vi "Fault_Abnormal_state.vi"() -> ()   [LabVIEW 2016]
panel:
  in  "e_MGCC_UnPlanISD_error":errorcluster
  in  "e_MGCC_PlanISD_error":errorcluster
  in  "Abnormal state flag":bool[](array[boolean])
  in  "Fault state flag":bool[](array[boolean])
  out "e_MGCC_StaEst_error":errorcluster[](array[cluster])
  out "e_MGCC_Resync_error":errorcluster[](array[cluster])
  out "e_MGCC_PQBal_error":errorcluster[](array[cluster])
  out "e_MGCC_PVFcst_error":errorcluster[](array[cluster])
  out "e_MGCC_ProtCoord_error":errorcluster[](array[cluster])
  out "e_MGCC_MdlMgmt_error":errorcluster
  out "e_MGCC_LoadFcst_error":errorcluster[](array[cluster])
  out "e_MGCC_Datalog_error":errorcluster[](array[cluster])
  out "e_MGCC_FntStaMach_error":errorcluster
  out "e_MGCC_EnergyMgmt_error":errorcluster[](array[cluster])
  out "e_MGCC_Commun_error":errorcluster[](array[cluster])
  out "e_MGCC_BlkStart_error":errorcluster[](array[cluster])
  out "Function enable by fault/abnormal":bool[][](array[boolean])
  out "Error State":errorcluster[](array[cluster])
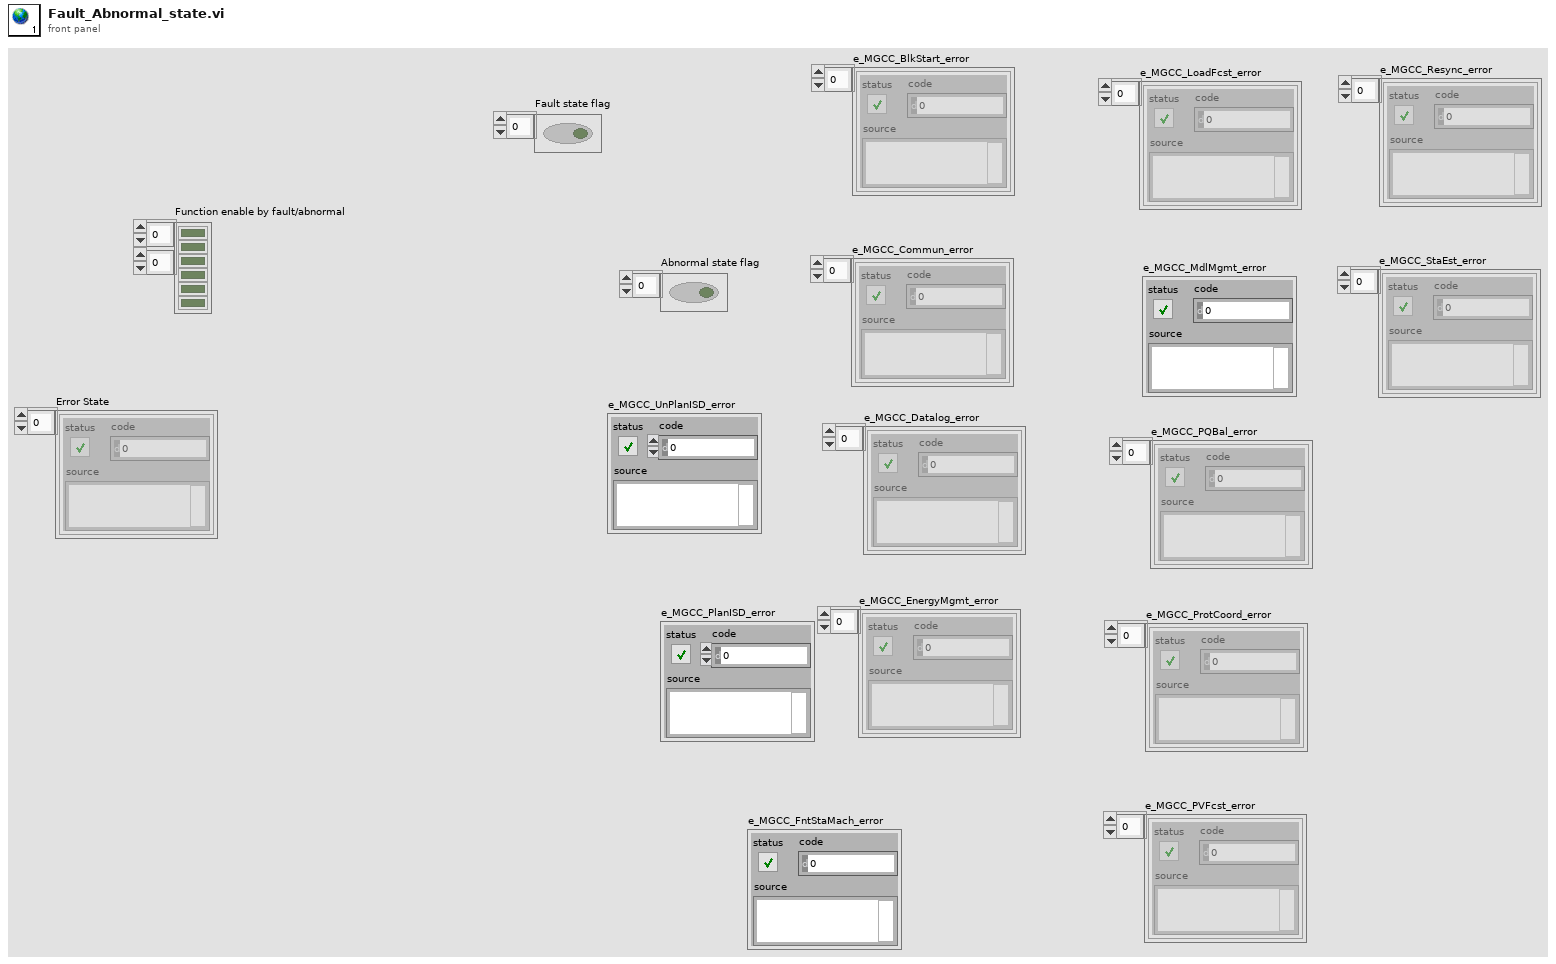
[diagram p1: front panel]
diagram:
